vi "ROS Init.vi"(6 "Cluster":cluster{"Topic to write":string, "type":string}={"Topic to write"="rio", "type"="std_msgs/Int32MultiArray"}, 10 "rosbridge port":u16, 11 "rosbridge server IP":string) -> (3 "output cluster":T1, 4 "Topic to write":string)   [LabVIEW 2015]
uses:
  <vilib>/Intelligent Energy/WebSockets API/WebSockets/WebSockets.lvlib
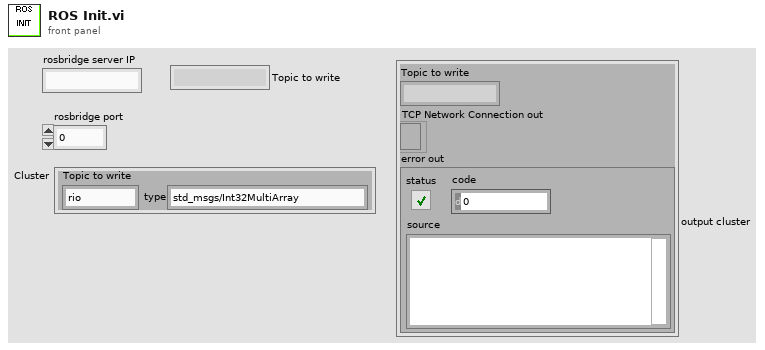
[diagram p1: front panel]
types:
  T1 = cluster{"Topic to write":string, "TCP Network Connection out":refnum<k5>, "error out":errorcluster}
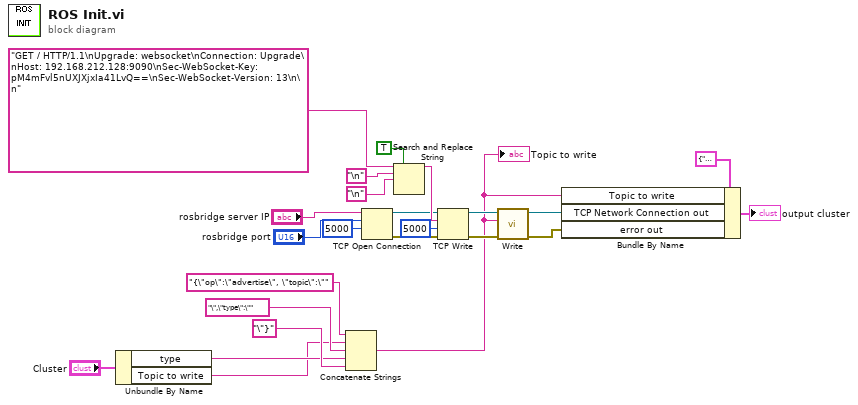
[diagram p0: block diagram]
diagram:
  n1 = Unbundle By Name("Cluster") -> ("type"=w9:string, "Topic to write"=w4:string)
  n2 = Concatenate Strings("{\"op\":\"advertise\", \"topic\":\"", w4, "\",\"type\":\"", w9, "\"}") -> (w3:string)
  "Topic to write" <- w3
  n3 = TCP Open Connection(address="rosbridge server IP", remote port or service name="rosbridge port", timeout ms (60000)=5000) -> (connection ID=w20:refnum<k5>, error out=w21:errorcluster)  [unwired: 2 in]
  n4 = Search and Replace String(replace all?=TRUE ("replace all? (F)"), input string="GET / HTTP/1.1\nUpgrade: websocket\nConnection: Upgrade\nHost: 192.168.212.128:9090\nSec-WebSocket-Key: pM4mFvl5nUXJXjxIa41LvQ==\nSec-WebSocket-Version: 13\n\n", search string="\n", replace string="\n") -> (result string=w22:string)  [unwired: 4 in, 3 out]
  n5 = TCP Write(connection ID=w20, data in=w22, error in (no error)=w21, 9:5000 ("timeout ms (25000)")) -> (connection ID out=w23:refnum<k5>, error out=w24:errorcluster)  [unwired: 1 out]
  n6 = call <vilib>:"Write.vi"("error in (no error)"=w24, "Data"=w3, "WebSocket Connection in"=w23) -> ("error out"=w6:errorcluster, "WebSocket Connection out"=w8:refnum<k5>)  [unwired: 7 in]
  n7 = Bundle By Name(cluster=T1 {"Topic to write"="", "TCP Network Connection out"=refnum, "error out"={"status"=FALSE, "code"=0, "source"=""}} ("input cluster"), "Topic to write"=w3, "TCP Network Connection out"=w8, "error out"=w6) -> (→"output cluster":T1)
